vi "SetCamMode.vi"(0 "Vision.lvlib:Vision.lvclass":refnum<class "Vision.lvclass">, 1 "Vision Processing?":bool, 3 "error in (no error)":errorcluster) -> (7 "Vision.lvlib:Vision.lvclass":refnum<class "Vision.lvclass">, 10 "error out":errorcluster)   [LabVIEW 2019, in "Vision.lvlib" / "Vision.lvclass"]
doc: "This VI changes the LED light mode and the camera mode to make the limelight usable for driver vision or computer vision."
uses:
  Vision.lvclass
  <vilib>/Rock Robotics/Network Tables/NT Write Number.vi
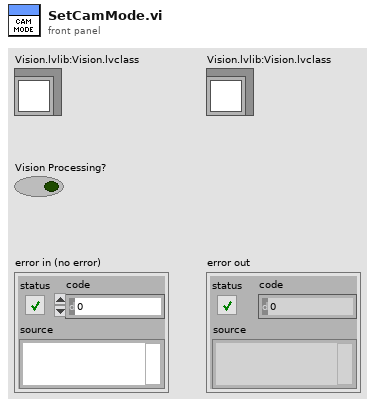
[diagram p1: front panel]
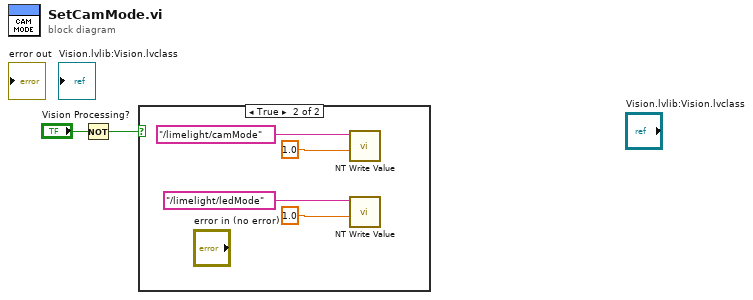
[diagram p0: block diagram]
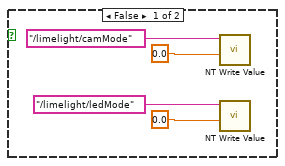
[diagram p2: hidden frame]
diagram:
  n1 = Not(x="Vision Processing?") -> (.not. x?=w1:bool)
  n2 = case shown="True" w1 {
    frame False {
      n3 = call-poly <vilib>:"NT Write Value.vi"("Numeric"=0.0, "Name"="/limelight/camMode") -> ()  [unwired: 9 in, 1 out]
      n4 = call-poly <vilib>:"NT Write Value.vi"("Numeric"=0.0, "Name"="/limelight/ledMode") -> ()  [unwired: 9 in, 1 out]
    }
    frame True {
      n5 = call-poly <vilib>:"NT Write Value.vi"("Numeric"=1.0, "Name"="/limelight/camMode") -> ()  [unwired: 9 in, 1 out]
      n6 = call-poly <vilib>:"NT Write Value.vi"("Numeric"=1.0, "Name"="/limelight/ledMode") -> ()  [unwired: 9 in, 1 out]
    }
  }
